vi "Test ATM Withdraw more than Balance Fails.vi"(8 "error in (no error)":errorcluster, 11 "Test Case In":refnum<class "Controller Test.lvclass">) -> (0 "error out":errorcluster, 3 "Test Case Out":refnum<class "Controller Test.lvclass">)   [LabVIEW 2020, in "Controller Test.lvclass"]
uses:
  Controller Test/Controller Test.lvclass
  C:/Program Files (x86)/National Instruments/LabVIEW 2020/vi.lib/Astemes/LUnit/Test Case.lvclass
  Account Database/Account Data.ctl
  ATM Controller/State.ctl
  <vilib>/Astemes/LUnit/Test Case.lvclass/Test Case.ctl
  01074fa8-ee8a-411d-bc8b-fc92c4f90959.vi
  1ace18d8-b683-4b1a-8a7a-31d11309c5eb.vi
  <vilib>/Astemes/LUnit/Palette/Pass.vi
  <vilib>/Astemes/LUnit/Palette/Fail.vi
  <vilib>/Astemes/LUnit/Compare Variants.vi
  <vilib>/Astemes/LUnit/Describe Comparison.vi
  <vilib>/Astemes/LUnit/Set Assertion Type.vi
  <vilib>/Astemes/LUnit/Add test result.vi
  <vilib>/Astemes/LUnit/Variant to string.vi
  <vilib>/Astemes/LUnit/LUnit Record Assertion Result.vi
  <vilib>/Astemes/LUnit/LUnit Aggregate Assertion Results.vi
  <vilib>/Astemes/LUnit/Method Result/LUnit Merge Status.vi
  <vilib>/Astemes/LUnit/LUnit Concatenate result strings.vi
  <vilib>/Utility/Data Type/Get Type Information.vi
  <vilib>/Utility/LVClass/Get LV Class Name.vi
  ATM Controller/ATM Controller.lvclass
  Account Database/Account Database.lvclass
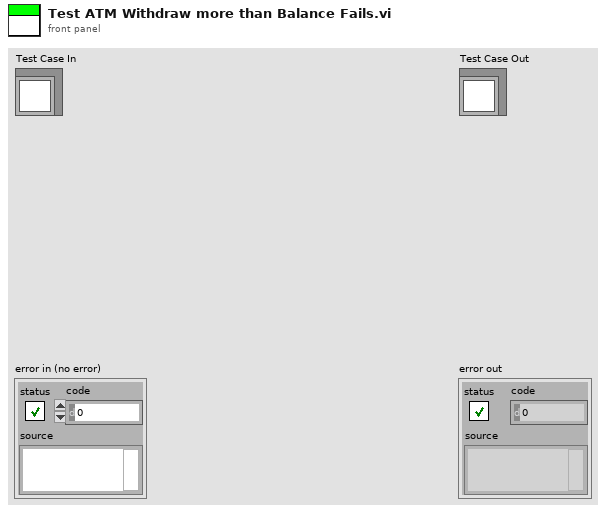
[diagram p1: front panel]
types:
  T1 = typedef "ATM Controller.lvclass/State.ctl" = enum16{"Start", "Card Inserted", "Verification Failed", "Verification Succeeded", "Depositing", "Depositing Completed", "Withdrawing", "Withdraw Completed", "Withdraw Failed", "Terminate"}
  T2 = typedef "Account Database.lvclass/Account Data.ctl" = cluster{"Account Number":string, "First Name":string, "Last Name":string, "Account Balance":string}
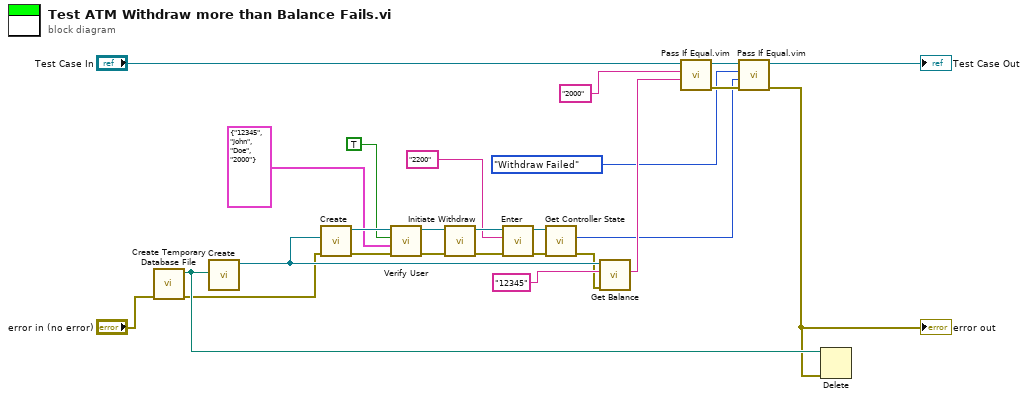
[diagram p0: block diagram]
diagram:
  n1 = call "Create Temporary Database File.vi"("error in (no error)"="error in (no error)") -> ("error out"=w2:errorcluster, "path"=w11:path)  [unwired: 9 in]
  n2 = call "Create.vi"("Data File"=w11) -> ("Account Database out"=w16:refnum<class "Account Database.lvclass">)  [unwired: 9 in, 1 out]
  n3 = call "Create.vi"("error in (no error)"=w2, "Account Database"=w16) -> ("error out"=w25:errorcluster, "ATM Controller out"=w20:refnum<class "ATM Controller.lvclass">)  [unwired: 8 in]
  n4 = call "Verify User.vi"("error in (no error)"=w25, "Account Data"=T2 {"Account Number"="12345", "First Name"="John", "Last Name"="Doe", "Account Balance"="2000"}, "Verified?"=TRUE, "ATM Controller in"=w20) -> ("error out"=w21:errorcluster, "ATM Controller out"=w19:refnum<class "ATM Controller.lvclass">)  [unwired: 6 in]
  n5 = call "Initiate Withdraw.vi"("error in (no error)"=w21, "ATM Controller in"=w19) -> ("error out"=w23:errorcluster, "ATM Controller out"=w24:refnum<class "ATM Controller.lvclass">)  [unwired: 8 in]
  n6 = call "Enter.vi"("error in (no error)"=w23, "User Input"="2200", "ATM Controller in"=w24) -> ("error out"=w14:errorcluster, "ATM Controller out"=w9:refnum<class "ATM Controller.lvclass">)  [unwired: 7 in]
  n7 = call "Get Controller State.vi"("error in (no error)"=w14, "ATM Controller in"=w9) -> ("error out"=w10:errorcluster, "ATM State"=w4:T1)  [unwired: 7 in, 1 out]
  n8 = call "Get Balance.vi"("error in (no error)"=w10, "Account Number"="12345", "Account Database in"=w16) -> ("Account Balance"=w13:string)  [unwired: 6 in, 2 out]
  n9 = call "Pass If Equal.vim"("Actual"=w13, "Expected"="2000" ("Account Balance"), "LUnit Test Case In"="Test Case In") -> ("error out"=w8:errorcluster, "LUnit Test Case Out"=w6:refnum<class "Controller Test.lvclass">)  [unwired: 7 in]
  n10 = call "Pass If Equal.vim"("error in (no error)"=w8, "Actual"=w4, "Expected"=State."Withdraw Failed" ("ATM State"), "LUnit Test Case In"=w6) -> ("error out"=w7:errorcluster, "LUnit Test Case Out"=→"Test Case Out":refnum<class "Controller Test.lvclass">)  [unwired: 6 in]
  "error out" <- w7
  n11 = Delete(path (use dialog)=w11, error in=w7) -> ()  [unwired: 3 in, 3 out]
